vi "Read Wheel Angle.vi"(2 "error in (no error)":errorcluster, 3 "Car.lvclass":refnum<class "Car.lvclass">) -> (0 "error out":errorcluster, 1 "Wheel Angle":dbl)   [LabVIEW 2015, in "Car.lvclass"]
uses:
  Car.lvclass
  Car.lvclass/Car.ctl
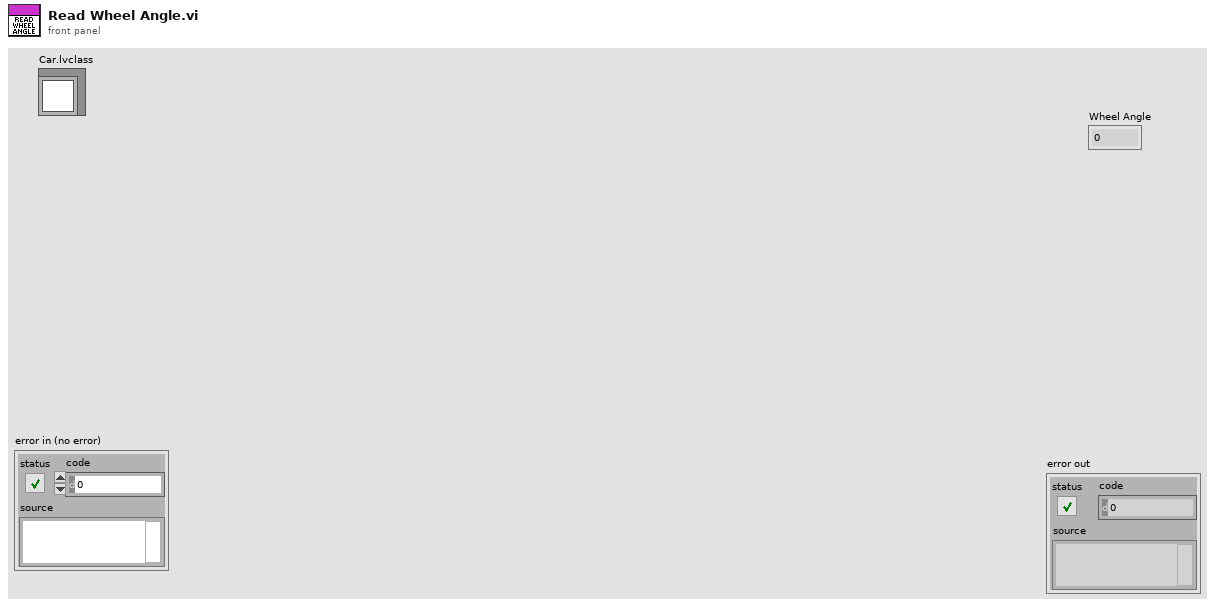
[diagram p1: front panel]
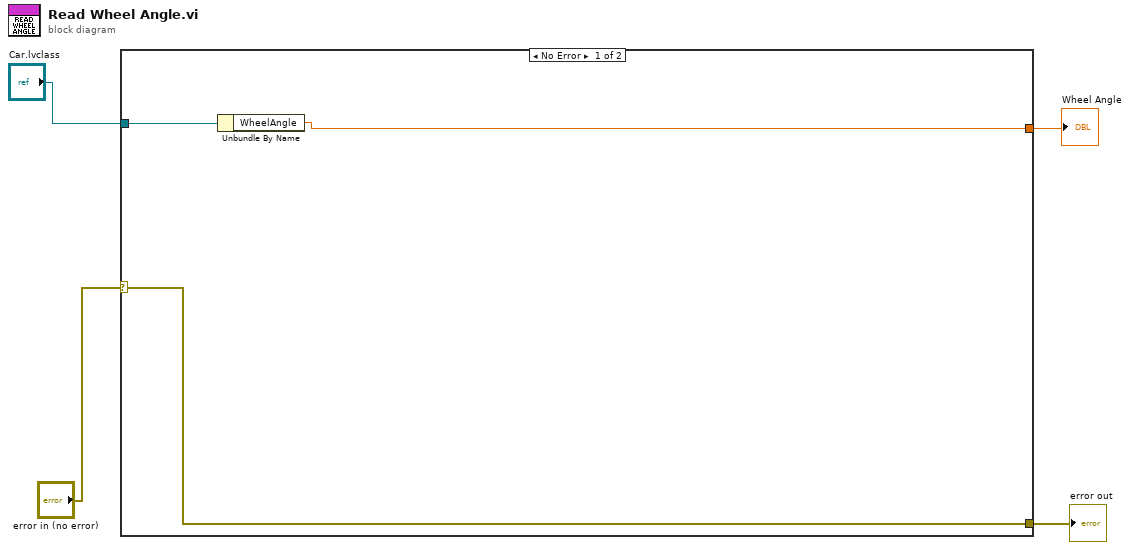
[diagram p0: block diagram]
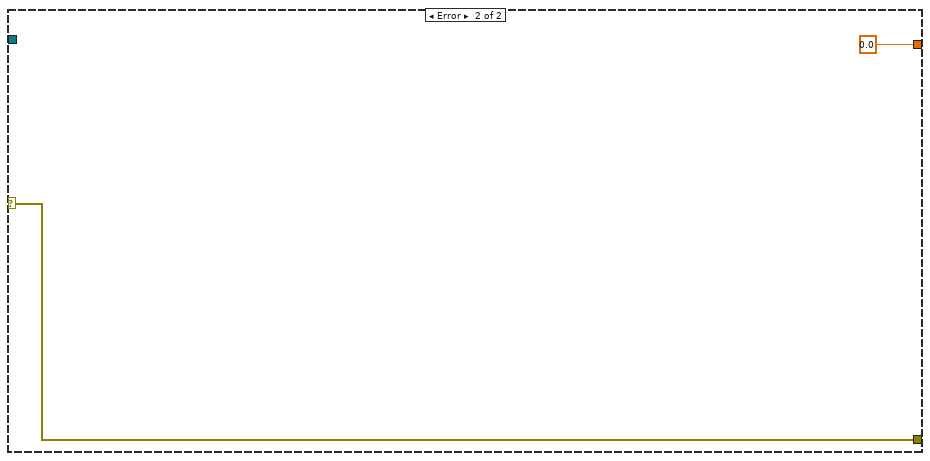
[diagram p2: hidden frame]
diagram:
  n1 = case shown="No Error" "error in (no error)" {
    selector: "error in (no error)" -> [w7 w9]
    tunnel: [w7 w9] -> w3
    tunnel: [w5 0.0] -> w2
    tunnel: "Car.lvclass" -> [w6 _]
    frame No Error {
      n2 = Unbundle By Name(w6) -> ("WheelAngle"=w5:dbl)
    }
    frame Error {
    }
  }
  "error out" <- w3
  "Wheel Angle" <- w2
